vi "GetPin.vi"(8 "error in (no error)":errorcluster, 9 "Pin":u8, 10 "Port":u8, 11 "Simulated Device in":refnum<class "Simulated Device.lvclass">) -> (0 "error out":errorcluster, 1 "Response":string, 2 "Value":bool, 3 "Simulated Device out":refnum<class "Simulated Device.lvclass">)   [LabVIEW 2020, in "Simulated Device.lvclass"]
doc: "Sends a command to read the pin status from the target device."
uses:
  Simulated Device.lvclass
  Controls/Device Code.ctl
  Controls/Device Command Code.ctl
  <vilib>/Utility/error.llb/Error Cluster From Error Code.vi
  <vilib>/ErrorRing/Error Ring.xnode
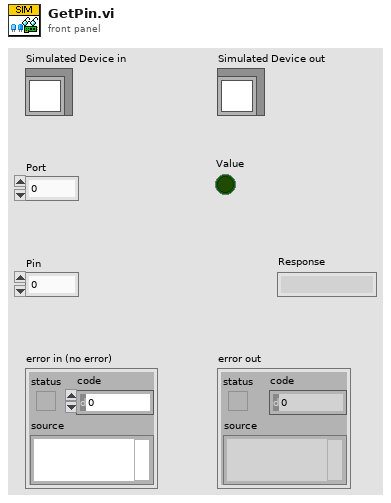
[diagram p1: front panel]
types:
  T1 = typedef "Device Command Code.ctl" = string
  T2 = typedef "Device Code.ctl" = string
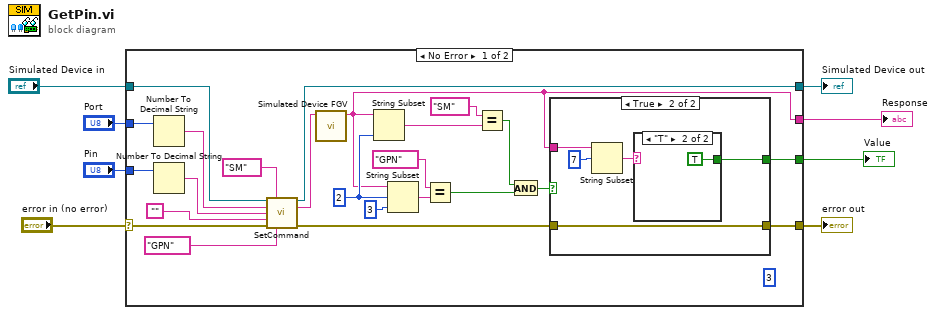
[diagram p0: block diagram]
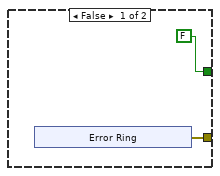
[diagram p2: hidden frame]
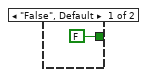
[diagram p3: hidden frame]
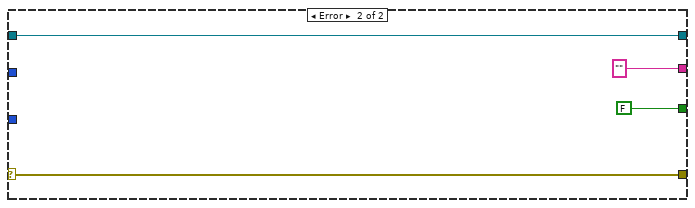
[diagram p4: hidden frame]
diagram:
  n1 = case shown="No Error" "error in (no error)" {
    selector: "error in (no error)" -> [w32 w49]
    tunnel: [w16 w49] -> w4
    tunnel: "Simulated Device in" -> [w30 w50]
    tunnel: [w23 w50] -> w7
    tunnel: "Port" -> [w28 _]
    tunnel: "Pin" -> [w26 _]
    tunnel: [w14 FALSE] -> w6
    tunnel: [w9 "" ("read buffer")] -> w5
    frame No Error {
      (unwired) 3 ("length (rest)")
      w21 = 2 ("length (rest)")
      n2 = Number To Decimal String(number=w28) -> (decimal integer string=w27:string)  [unwired: 1 in]
      n3 = Number To Decimal String(number=w26) -> (decimal integer string=w25:string)  [unwired: 1 in]
      n4 = call-dynamic "SetCommand.vi"("Simulated Device in"=w30, "Device Code"=T2 "SM", "Parameter 1"=w27, "Parameter 2"=w25, "Parameter 3"="", "error in (no error)"=w32, "Command Code"=T1 "GPN") -> ("Simulated Device out"=w23:refnum<class "Simulated Device.lvclass">, "Command"=w10:string, "error out"=w11:errorcluster)  [unwired: 6 in]
      n5 = call "Simulated Device FGV.vi"("Request"=w10) -> ("Response"=w9:string)  [unwired: 10 in]
      n6 = String Subset(string=w9, length (rest)=w21) -> (substring=w13:string)  [unwired: 1 in]
      n7 = String Subset(string=w9, offset (0)=w21, length (rest)=3 ("length (rest)")) -> (substring=w22:string)
      n8 = Equal?(x=T1 "GPN" ("Command Code"), y=w22) -> (x = y?=w18:bool)
      n9 = Equal?(x=T2 "SM" ("Device Code"), y=w13) -> (x = y?=w15:bool)
      n10 = And(x=w15, y=w18) -> (x .and. y?=w17:bool)
      n11 = case shown="True" w17 {
        tunnel: w11 -> [_ w44]
        tunnel: [w34 w44] -> w16
        tunnel: w9 -> [_ w43]
        tunnel: [FALSE w40] -> w14
        frame False {
          n12 = xnode "Error Ring"() -> ("error out"=w34:errorcluster)
        }
        frame True {
          n13 = String Subset(string=w43, offset (0)=7) -> (substring=w41:string)  [unwired: 1 in]
          n14 = case shown="\"T\"" w41 {
            tunnel: [FALSE TRUE] -> w40
            frame "False", Default {
            }
            frame "T" {
            }
          }
        }
      }
    }
    frame Error {
    }
  }
  "error out" <- w4
  "Simulated Device out" <- w7
  "Response" <- w5
  "Value" <- w6
